vi "FP Cleanup.vi"(8 "error in":errorcluster, 11 "vi refnum":refnum<vi>) -> (0 "error out":errorcluster, 3 "vi refnum out":refnum<vi>)   [LabVIEW 2021, in "MeasurementClient Editor.lvlib"]
uses:
  MeasurementClient Editor.lvlib
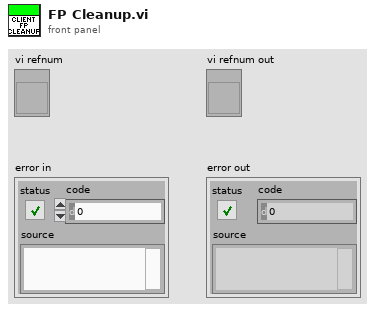
[diagram p1: front panel]
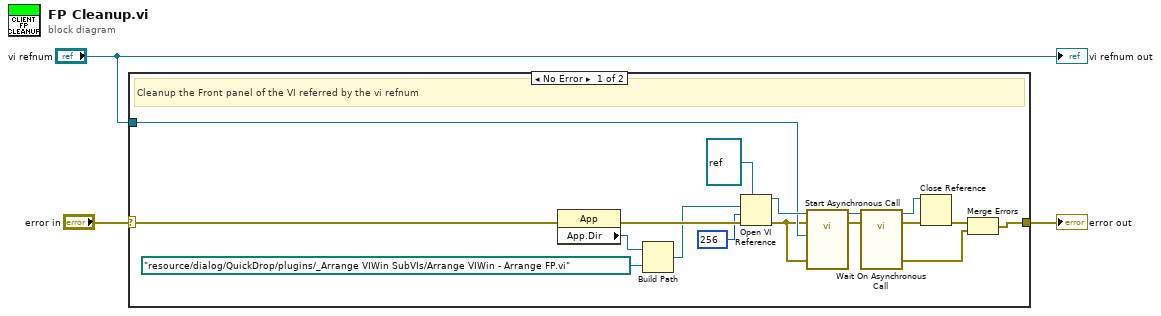
[diagram p0: block diagram]
diagram:
  n1 = case shown="No Error" "error in" {
    selector: "error in" -> [w20 w21]
    tunnel: [w8 w21] -> w3
    tunnel: "vi refnum" -> [w12 _]
    frame No Error {
      # "Cleanup the Front panel of the VI referred by the vi refnum"
      n2 = property class="App"(error in=w20) -> (error out=w19:errorcluster, "App.Dir"=w17:path)  [unwired: 1 in, 1 out]
      n3 = Build Path(base path=w17, name or relative path=path "resource/dialog/QuickDrop/plugins/_Arrange VIWin SubVIs/Arrange VIWin - Arrange FP.vi") -> (appended path=w4:path)
      n4 = Open VI Reference(type specifier VI Refnum (for type only)=refnum<vi> refnum, vi path=w4, options=256, error in (no error)=w19) -> (vi reference=w13:refnum<vi>, error out=w11:errorcluster)  [unwired: 2 in]
      n5 = call-by-ref "Start Asynchronous Call"(reference=w13, error in=w11, "VI"=w12, "error in"=w11) -> (reference out=w9:refnum<vi>, error out=w14:errorcluster)  [unwired: 13 in, 1 out]
      n6 = call-by-ref "Wait On Asynchronous Call"(reference=w9, error in=w14) -> (reference out=w5:refnum<vi>, error out=w10:errorcluster, 15:"error out"=w7:errorcluster)  [unwired: 15 in]
      n7 = Close Reference(reference=w5, error in (no error)=w10) -> (error out=w6:errorcluster)
      n8 = Merge Errors(w6, w7) -> (w8:errorcluster)
    }
    frame Error {
      # "Pass"
    }
  }
  "error out" <- w3
  "vi refnum out" <- "vi refnum"
